vi "ConfigureDlg.vi"(8 "error in (no error)":errorcluster, 11 "C37.118 PMU in":refnum<class "C37.118 Sim.lvclass">) -> (0 "error out":errorcluster, 2 "Changed":bool, 3 "C37.118 PMU out":refnum<class "C37.118 Sim.lvclass">)   [LabVIEW 2018, in "SensorPlugins.lvlib" / "C37.118 Sim.lvclass"]
uses:
  C37.118 Sim.lvclass
  C:/projects/ICDAS/NistPluggableModules/Sensor/SensorPlugins/PmuBaseClass/PmuBase.lvclass
  C:/Program Files/National Instruments/LabVIEW 2018/user.lib/NIST/BaseClasses/BasePlugin_class/BasePlugin.lvclass
  PmuBaseClass/Typedef/PmuConfig.ctl
  PmuBaseClass/Typedef/ePhases.ctl
  PmuBaseClass/PmuBase.lvclass/PmuBase.ctl
  C37.118 Sim.lvclass/C37.118 Sim.ctl
  <userlib>/NIST/BaseClasses/BasePlugin_class/BasePlugin.lvclass/BasePlugin.ctl
  FGen/MemberClasses/FunctionBaseClass/FunctionBase.lvclass
  PmuBaseClass/Accessors/Read PmuConfig.vi
  PmuBaseClass/Accessors/Read PhaseArray.vi
  Accessors/Read Time.vi
  Accessors/Read FunctionIniFilePath.vi
  PmuBaseClass/Accessors/Write PmuConfig.vi
  PmuBaseClass/Accessors/Write PhaseArray.vi
  Accessors/Write Time.vi
  <userlib>/NIST/BaseClasses/BasePlugin_class/Accessors/Read PluginIniFilePath.vi
  <userlib>/NIST/BaseClasses/BasePlugin_class/Accessors/Write PluginIniFilePath.vi
  Accessors/Write Function.vi
  Accessors/Write FunctionIniFilePath.vi
  Accessors/Read Function.vi
  <vilib>/Utility/error.llb/Error Cluster From Error Code.vi
  <vilib>/ErrorRing/Error Ring.xnode
  <vilib>/Utility/config.llb/NI_LVConfig.lvlib
  <userlib>/NIST/NISTErrorLib/NISTErrorLib.lvlib
  <userlib>/NIST/BaseClasses/Object_class/BaseObject.lvclass
  PmuBaseClass/PmuBase.lvclass
panel:
  in  "Duration (s)":dbl
  in  "btnSaveAs":bool
  in  "FunctionIniFilePath":path
  in  "btnFuncConfig":bool
  in  "btnCancel":bool
  in  "BtnDone":bool
  in  "PhaseArray":T1[](array[typedef])=[enum."VA", enum."VB", enum."VC", enum."V+", enum."IA", enum."IB", enum."IC", enum."I+"]
  in  "PmuConfig":T2={"Class"=enum."M", "Fs"=60, "F0"=60, "FSamp"=60, "SettlingTime"=0.0, "T0"=0.0}
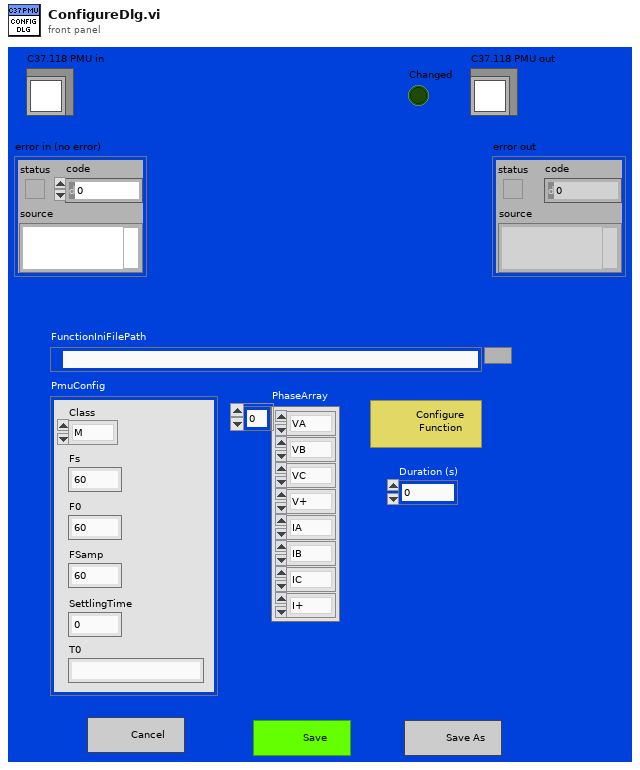
[diagram p1: front panel]
types:
  T1 = typedef "SensorPlugins.lvlib/PmuBase.lvclass/ePhases.ctl" = enum16{"VA", "VB", "VC", "V+", "IA", "IB", "IC", "I+", "none"}
  T2 = typedef "SensorPlugins.lvlib/PmuBase.lvclass/PmuConfig.ctl" = cluster{"Class":enum16{"M", "P"}, "Fs":i32, "F0":i32, "FSamp":i32, "SettlingTime":dbl, "T0":ext}
  T3 = enum8{"Enabled", "Disabled", "Disabled and Grayed Out"}
  T4 = enum32{"Invalid", "Standard", "Closed", "Hidden", "Minimized", "Maximized"}
  T5 = enum32{"Invalid", "Default", "Floating", "Floating/Auto-Hide", "Modal"}
  T6 = typedef "NI_LVConfig.lvlib/Config Data RefNum.ctl" = refnum<k1>
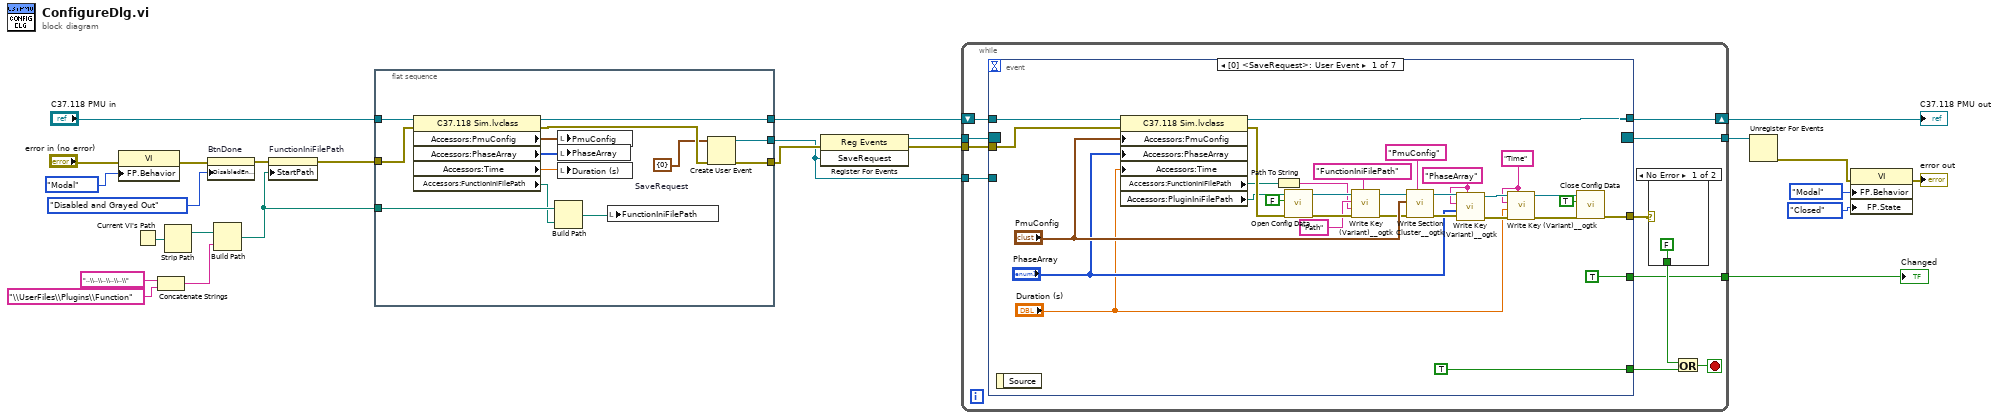
[diagram p0: block diagram]
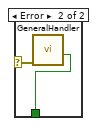
[diagram p2: hidden frame]
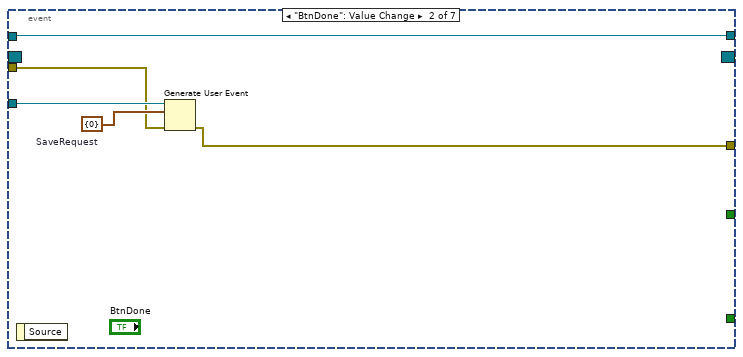
[diagram p3: hidden frame]
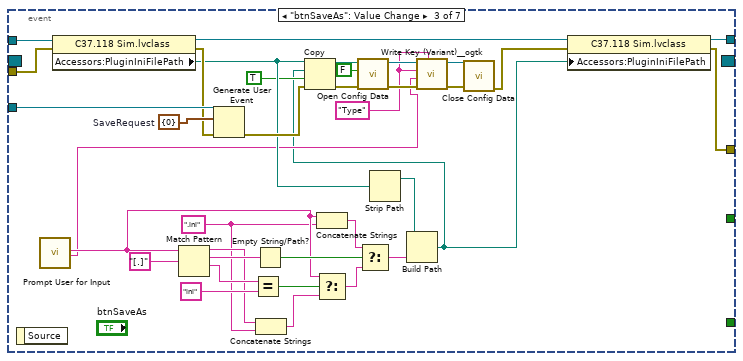
[diagram p4: hidden frame]
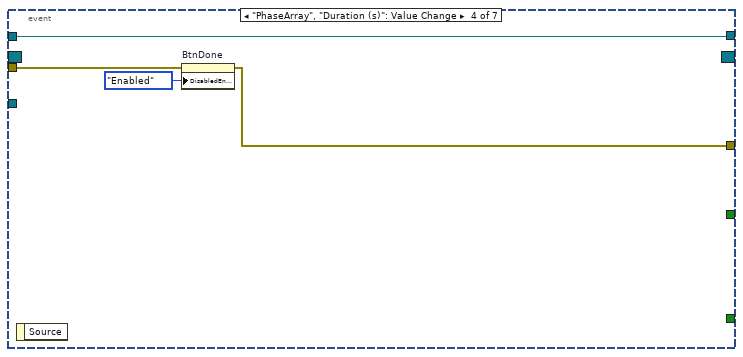
[diagram p5: hidden frame]
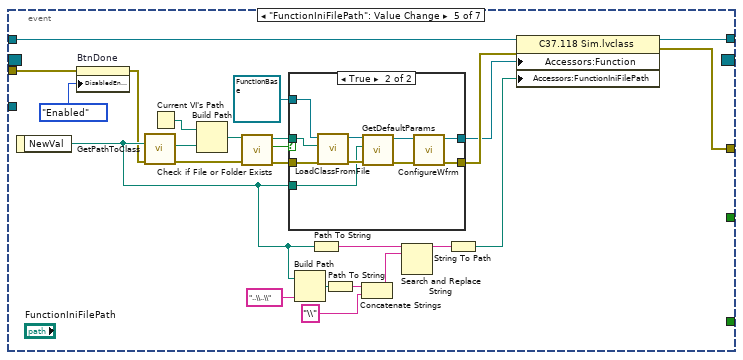
[diagram p6: hidden frame]
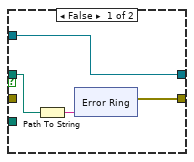
[diagram p7: hidden frame]
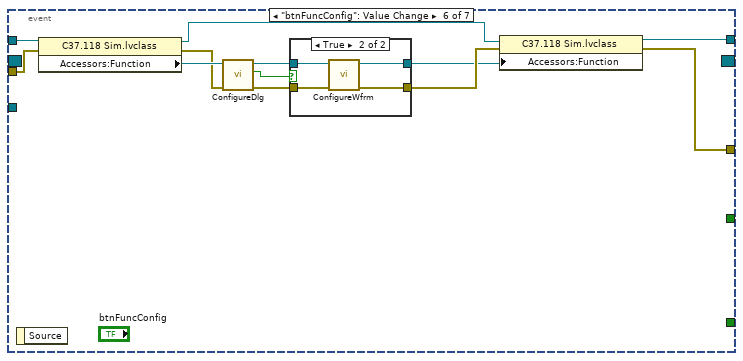
[diagram p8: hidden frame]
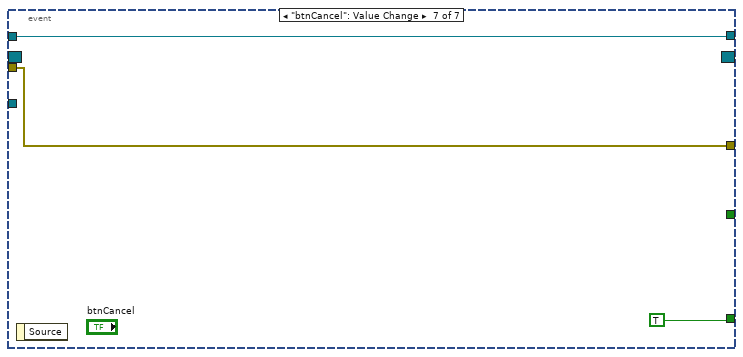
[diagram p10: hidden frame]
diagram:
  n1 = property class="VI"(error in="error in (no error)", "FP.Behavior"=T5."Modal" ("Front Panel Window:Behavior")) -> (error out=w16:errorcluster)  [unwired: 1 in, 1 out]
  n2 = Current VI's Path() -> (path=w11:path)
  n3 = Concatenate Strings("..\\..\\..\\..\\..\\", "\\UserFiles\\Plugins\\Function" ("name or relative path")) -> (w13:string)
  n4 = Strip Path(path=w11) -> (stripped path=w14:path)  [unwired: 1 out]
  n5 = property on="BtnDone" class="Bool"(error in=w16, "DisabledEnum"=T3."Disabled and Grayed Out" ("Disabled")) -> (error out=w9:errorcluster)  [unwired: 1 in, 1 out]
  n6 = Build Path(base path=w14, name or relative path=w13) -> (appended path=w7:path)
  n7 = property on="FunctionIniFilePath" class="Path"(error in=w9, "StartPath"=w7) -> (error out=w8:errorcluster)  [unwired: 1 in, 1 out]
  n8 = flat-sequence {
    tunnel: "C37.118 PMU in" -> [w38]
    tunnel: [w37] -> w23
    tunnel: [w31] -> w6
    tunnel: w8 -> [w36]
    tunnel: w7 -> [w33]
    tunnel: [w28] -> w4
    frame #0 {
      w29 = cluster{"Num":i32} {"Num"=0}  # SaveRequest
      n9 = property class="C37.118 Sim.lvclass"(reference=w38, error in=w36) -> (reference out=w37:refnum<class "C37.118 Sim.lvclass">, error out=w30:errorcluster, "Accessors:PmuConfig"=w35:T2, "Accessors:PhaseArray"=w34:T1[], "Accessors:Time"=w26:ext, "Accessors:FunctionIniFilePath"=w27:path)
      n10 = Build Path(base path=w33, name or relative path=w27) -> (appended path=w32:path)
      n11 = local write "PmuConfig"(w35) -> ()
      n12 = local write "PhaseArray"(w34) -> ()
      n13 = local write "Duration (s)"(w26) -> ()
      n14 = local write "FunctionIniFilePath"(w32) -> ()
      n15 = Create User Event(user event datatype=w29, error in=w30) -> (user event=w28:refnum<user-event>, error out=w31:errorcluster)
    }
  }
  n16 = register-events(error in=w6, w4) -> (reference out=w3:refnum<event-registration>, error out=w5:errorcluster)  [unwired: 1 in]
  n17 = while {
    shift-right: [w47] -> w24
    shift-left: w23 -> [w49]
    tunnel: w5 -> [w48]
    tunnel: [w42] -> w21
    tunnel: w4 -> [w41]
    tunnel: w3 -> [w40]
    tunnel: [w39] -> w2
    stop <- w43 stop-if-true
    n18 = event shown="[0] <SaveRequest>: User Event" {
      selector: w40 -> [_ _ _ _ _ _ _]
      dyn-events: [_ _ _ _ _ _ _] -> w39
      timeout: _ -> [_ _ _ _ _ _ _]
      tunnel: w49 -> [w82 w83 w111 w126 w137 w185 w194]
      tunnel: w48 -> [w80 w85 w108 w127 w130 w184 w193]
      tunnel: [w69 w84 w89 w124 w131 w179 w193] -> w44
      tunnel: [TRUE _ _ _ _ _ TRUE] -> w46
      tunnel: [w79 w83 w109 w126 w132 w180 w194] -> w47
      tunnel: [TRUE _ _ _ _ _ _] -> w42
      tunnel: w41 -> [_ w87 w107 _ _ _ _]
      event User Event {
        w58 = "Time" ("section")
        w68 = "PhaseArray" ("section (optional)")
        n19 = event-data() -> ()  [unwired: 1 in, 1 out]
        n20 = property class="C37.118 Sim.lvclass"(reference=w82, error in=w80, "Accessors:PmuConfig"="PmuConfig", "Accessors:PhaseArray"="PhaseArray", "Accessors:Time"="Duration (s)") -> (reference out=w79:refnum<class "C37.118 Sim.lvclass">, error out=w77:errorcluster, "Accessors:FunctionIniFilePath"=w54:path, "Accessors:PluginIniFilePath"=w66:path)
        n21 = Path To String(path=w54) -> (string=w53:string)
        n22 = call <vilib>:"Open Config Data.vi"("error in (no error)"=w77, "create file if necessary (T)"=FALSE, "configuration file path"=w66) -> ("error out"=w64:errorcluster, "refnum"=w76:T6)  [unwired: 6 in, 1 out]
        n23 = call <userlib>:"Write Key (Variant)__ogtk.vi"("section"="FunctionIniFilePath", "error in (no error)"=w64, "key-value"=w53, "key (optional)"="Path", "refnum"=w76) -> ("error out"=w63:errorcluster, "refnum out"=w65:T6)  [unwired: 5 in]
        n24 = call <userlib>:"Write Section Cluster__ogtk.vi"("section (optional)"="PmuConfig", "error in (no error)"=w63, "Section Formatted Cluster"="PmuConfig", "refnum"=w65) -> ("error out"=w73:errorcluster, "dup refnum"=w72:T6)  [unwired: 6 in]
        n25 = call <userlib>:"Write Key (Variant)__ogtk.vi"("section"=w68, "error in (no error)"=w73, "key-value"="PhaseArray", "key (optional)"=w68, "refnum"=w72) -> ("error out"=w60:errorcluster, "refnum out"=w59:T6)  [unwired: 5 in]
        n26 = call <userlib>:"Write Key (Variant)__ogtk.vi"("section"=w58, "error in (no error)"=w60, "key-value"="Duration (s)", "key (optional)"=w58, "refnum"=w59) -> ("error out"=w57:errorcluster, "refnum out"=w56:T6)  [unwired: 5 in]
        n27 = call <vilib>:"Close Config Data.vi"("error in (no error)"=w57, "write file if changed (T)"=TRUE, "refnum"=w56) -> ("error out"=w69:errorcluster)  [unwired: 7 in, 1 out]
      }
      event "BtnDone": Value Change {
        w86 = cluster{"Num":i32} {"Num"=0}  # SaveRequest
        n28 = event-data() -> ()  [unwired: 1 in, 1 out]
        n29 = Generate User Event(user event=w87, event data cluster=w86, error in=w85) -> (error out=w84:errorcluster)  [unwired: 1 in, 1 out]
      }
      event "btnSaveAs": Value Change {
        w88 = "Type"
        w106 = cluster{"Num":i32} {"Num"=0}  # SaveRequest
        w92 = ".ini" ("string")
        n30 = event-data() -> ()  [unwired: 1 in, 1 out]
        n31 = call "Prompt User for Input"() -> ("File Name"=w112:string, "PluginType Name"=w93:string)  [unwired: 16 in, 2 out]
        n32 = property class="C37.118 Sim.lvclass"(reference=w111, error in=w108) -> (reference out=w110:refnum<class "C37.118 Sim.lvclass">, error out=w105:errorcluster, "Accessors:PluginIniFilePath"=w96:path)
        n33 = Match Pattern(string=w112, regular expression="[.]" ("string")) -> (before substring=w119:string, match substring=w121:string, after substring=w122:string)  [unwired: 1 in, 1 out]
        n34 = Generate User Event(user event=w107, event data cluster=w106, error in=w105) -> (error out=w97:errorcluster)  [unwired: 1 in, 1 out]
        n35 = Equal?(x=w122, y="ini" ("string")) -> (x = y?=w118:bool)
        n36 = Empty String/Path?(string/path=w121) -> (empty?=w116:bool)
        n37 = Concatenate Strings(w119, w92) -> (w117:string)
        n38 = Concatenate Strings(w112, w92) -> (w114:string)
        n39 = Select(t=w112, s=w118, f=w117) -> (s? t:f=w115:string)
        n40 = Select(t=w114, s=w116, f=w115) -> (s? t:f=w113:string)
        n41 = Strip Path(path=w96) -> (stripped path=w95:path)  [unwired: 1 out]
        n42 = Build Path(base path=w95, name or relative path=w113) -> (appended path=w91:path)
        n43 = Copy(8:w97, 9:TRUE ("overwrite (F)"), 10:w91, 11:w96) -> (0:w98:errorcluster, 3:w99:path)  [unwired: 1 in, 1 out]
        n44 = call <vilib>:"Open Config Data.vi"("error in (no error)"=w98, "create file if necessary (T)"=FALSE, "configuration file path"=w99) -> ("error out"=w101:errorcluster, "refnum"=w102:T6)  [unwired: 6 in, 1 out]
        n45 = call <userlib>:"Write Key (Variant)__ogtk.vi"("section"=w88, "error in (no error)"=w101, "key-value"=w93, "key (optional)"=w88, "refnum"=w102) -> ("error out"=w103:errorcluster, "refnum out"=w104:T6)  [unwired: 5 in]
        n46 = call <vilib>:"Close Config Data.vi"("error in (no error)"=w103, "refnum"=w104) -> ("error out"=w90:errorcluster)  [unwired: 8 in, 1 out]
        n47 = property class="C37.118 Sim.lvclass"(reference=w110, error in=w90, "Accessors:PluginIniFilePath"=w91) -> (reference out=w109:refnum<class "C37.118 Sim.lvclass">, error out=w89:errorcluster)
      }
      event "PhaseArray", "Duration (s)": Value Change {
        n48 = event-data() -> ()  [unwired: 1 in, 1 out]
        n49 = property on="BtnDone" class="Bool"(error in=w127, "DisabledEnum"=T3."Enabled" ("Disabled")) -> (error out=w124:errorcluster)  [unwired: 1 in, 1 out]
      }
      event "FunctionIniFilePath": Value Change {
        n50 = event-data() -> ("NewVal"=w138:path)  [unwired: 1 in]
        n51 = property on="BtnDone" class="Bool"(error in=w130, "DisabledEnum"=T3."Enabled" ("Disabled")) -> (error out=w129:errorcluster)  [unwired: 1 in, 1 out]
        n52 = call <userlib>:"GetPathToClass.vi"("error in (no error)"=w129, "configuration file path"=w138) -> ("error IO"=w149:errorcluster, "PathToClass"=w152:path)  [unwired: 8 in]
        n53 = Current VI's Path() -> (path=w151:path)
        n54 = Build Path(base path=w151, name or relative path=w152) -> (appended path=w150:path)
        n55 = call <vilib>:"Check if File or Folder Exists.vi"("error in (no error)"=w149, "path"=w150) -> ("error out"=w146:errorcluster, "file or folder exists?"=w148:bool, "dup path"=w147:path)  [unwired: 7 in]
        n56 = case shown="True" w148 {
          tunnel: w147 -> [w155 w173]
          tunnel: w146 -> [_ w171]
          tunnel: refnum<class "FunctionBase.lvclass"> refnum ("Functions.lvlib:FunctionBase.lvclass") -> [w153 w172]
          tunnel: w138 -> [_ w168]
          tunnel: [w154 w167] -> w136
          tunnel: [w153 w166] -> w135
          frame False {
            n57 = Path To String(path=w155) -> (string=w156:string)
            n58 = xnode "Error Ring"("parameter 0"=w156) -> ("error out"=w154:errorcluster)
          }
          frame True {
            n59 = call-dynamic "LoadClassFromFile.vi"("error in (no error)"=w171, "class path"=w173, "reference in"=w172) -> ("error out"=w170:errorcluster, "reference out"=w169:refnum<class "FunctionBase.lvclass">)  [unwired: 7 in]
            n60 = call-dynamic "GetDefaultParams.vi"("error in (no error)"=w170, "Path"=w168, "FunctionBase in"=w169) -> ("error out"=w164:errorcluster, "FunctionBase out"=w165:refnum<class "FunctionBase.lvclass">)  [unwired: 7 in]
            n61 = call-dynamic "ConfigureWfrm.vi"("error in (no error)"=w164, "FunctionBase in"=w165) -> ("error out"=w167:errorcluster, "FunctionBase out"=w166:refnum<class "FunctionBase.lvclass">)  [unwired: 8 in]
          }
        }
        n62 = Build Path(base path=w138, name or relative path="..\\..\\") -> (appended path=w142:path)
        n63 = Path To String(path=w138) -> (string=w143:string)
        n64 = Path To String(path=w142) -> (string=w141:string)
        n65 = Concatenate Strings(w141, "\\" ("string")) -> (w139:string)
        n66 = Search and Replace String(input string=w143, search string=w139) -> (result string=w134:string)  [unwired: 6 in, 3 out]
        n67 = String To Path(string=w134) -> (path=w133:path)
        n68 = property class="C37.118 Sim.lvclass"(reference=w137, error in=w136, "Accessors:Function"=w135, "Accessors:FunctionIniFilePath"=w133) -> (reference out=w132:refnum<class "C37.118 Sim.lvclass">, error out=w131:errorcluster)
      }
      event "btnFuncConfig": Value Change {
        n69 = event-data() -> ()  [unwired: 1 in, 1 out]
        n70 = property class="C37.118 Sim.lvclass"(reference=w185, error in=w184) -> (reference out=w181:refnum<class "C37.118 Sim.lvclass">, error out=w182:errorcluster, "Accessors:Function"=w183:refnum<class "FunctionBase.lvclass">)
        n71 = call-dynamic "ConfigureDlg.vi"("error in (no error)"=w182, "FunctionBase in"=w183) -> ("error out"=w177:errorcluster, "Changed"=w174:bool, "FunctionBase out"=w178:refnum<class "FunctionBase.lvclass">)  [unwired: 7 in]
        n72 = case shown="True" w174 {
          tunnel: w178 -> [w187 w191]
          tunnel: w177 -> [w186 w190]
          tunnel: [w186 w189] -> w176
          tunnel: [w187 w188] -> w175
          frame False {
          }
          frame True {
            n73 = call-dynamic "ConfigureWfrm.vi"("error in (no error)"=w190, "FunctionBase in"=w191) -> ("error out"=w189:errorcluster, "FunctionBase out"=w188:refnum<class "FunctionBase.lvclass">)  [unwired: 8 in]
          }
        }
        n74 = property class="C37.118 Sim.lvclass"(reference=w181, error in=w176, "Accessors:Function"=w175) -> (reference out=w180:refnum<class "C37.118 Sim.lvclass">, error out=w179:errorcluster)
      }
      event "btnCancel": Value Change {
        n75 = event-data() -> ()  [unwired: 1 in, 1 out]
      }
    }
    n76 = case shown="No Error" w44 {
      selector: w44 -> [_ w51]
      tunnel: [FALSE ("Stop") w52] -> w45
      frame No Error {
      }
      frame Error {
        n77 = call <userlib>:"GeneralHandler.vi"("error in (no error)"=w51) -> ("Stop"=w52:bool)  [unwired: 6 in, 4 out]
      }
    }
    n78 = Or(x=w45, y=w46) -> (x .or. y?=w43:bool)
  }
  "C37.118 PMU out" <- w24
  "Changed" <- w21
  n79 = Unregister For Events(event registration refnum=w2) -> (error out=w1:errorcluster)  [unwired: 1 in]
  n80 = property class="VI"(error in=w1, "FP.Behavior"=T5."Modal" ("Front Panel Window:Behavior"), "FP.State"=T4."Closed" ("Front Panel Window:State")) -> (error out=→"error out":errorcluster)  [unwired: 1 in, 1 out]
